vi "Test MQTT-3.1.3-4.vi"(8 "error in (no error)":errorcluster) -> (0 "error out":errorcluster)   [LabVIEW 2013]
uses:
  <vilib>/LabVIEW Open Source Project/MQTT Control Packets/Control Packets/ControlPacket/ControlPacket.lvclass/ControlPacket.ctl
  <vilib>/addons/_JKI Toolkits/Caraya/classes/Assert/Assert Greater_Variant.vi
  <vilib>/LabVIEW Open Source Project/MQTT Control Packets/Control Packets/CONNECT/CONNECT.lvclass
  <vilib>/addons/_JKI Toolkits/Caraya/classes/Test/Test.lvclass
  <vilib>/addons/_JKI Toolkits/Caraya/classes/Assert/Assert.lvclass
  <vilib>/LabVIEW Open Source Project/MQTT Control Packets/Control Packets/ControlPacket/ControlPacket.lvclass
panel:
  out "size(s) 2":i32
  out "size(s)":i32
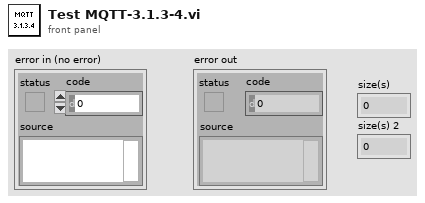
[diagram p1: front panel]
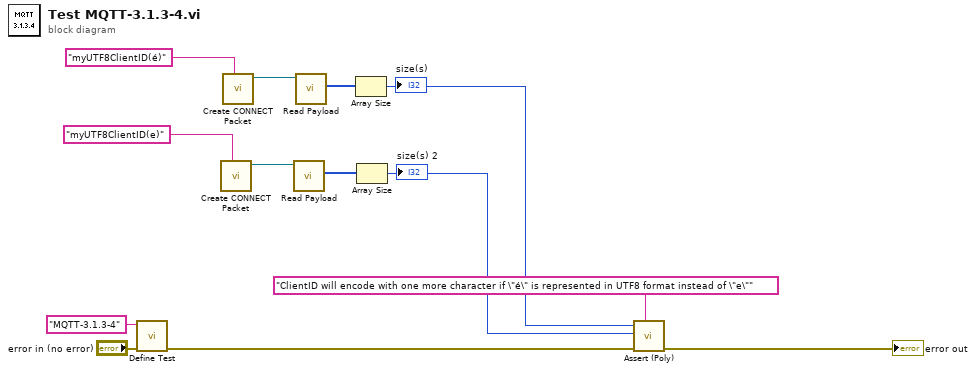
[diagram p0: block diagram]
diagram:
  n1 = call <vilib>:"Define Test.vi"("error in (no error)"="error in (no error)", "Label (VI Title)"="MQTT-3.1.3-4") -> ("error out"=w10:errorcluster)  [unwired: 9 in]
  n2 = call <vilib>:"Create CONNECT Packet.vi"("Client ID (empty: generate new)"="myUTF8ClientID(e)") -> ("CONNECT"=w8:refnum<class "CONNECT.lvclass">)  [unwired: 8 in, 2 out]
  n3 = call <vilib>:"Create CONNECT Packet.vi"("Client ID (empty: generate new)"="myUTF8ClientID(é)") -> ("CONNECT"=w6:refnum<class "CONNECT.lvclass">)  [unwired: 8 in, 2 out]
  n4 = call <vilib>:"Read Payload.vi"("ControlPacket in"=w8) -> ("Payload"=w4:u8[])  [unwired: 9 in, 1 out]
  n5 = call <vilib>:"Read Payload.vi"("ControlPacket in"=w6) -> ("Payload"=w5:u8[])  [unwired: 9 in, 1 out]
  n6 = Array Size(array=w5) -> (size(s)=w2:i32)
  "size(s)" <- w2
  n7 = Array Size(array=w4) -> (size(s)=w1:i32)
  "size(s) 2" <- w1
  n8 = call-poly <vilib>:"Assert (Poly).vi"("Label"="ClientID will encode with one more character if \"é\" is represented in UTF8 format instead of \"e\"", "error in (no error)"=w10, "Y"=w1, "X"=w2) -> ("error out"=→"error out":errorcluster)  [unwired: 7 in]
